vi "Read Coords.vi"(8 "error in (no error)":errorcluster, 11 "ShortcutMenuSelectionMsg in":refnum<class "ShortcutMenuSelectionMsg.lvclass">) -> (0 "error out":errorcluster, 2 "Coords":T1, 3 "ShortcutMenuSelectionMsg out":refnum<class "ShortcutMenuSelectionMsg.lvclass">)   [LabVIEW 2015, in "ActorEvents.lvlib" / "ShortcutMenuSelectionMsg.lvclass"]
uses:
  ShortcutMenuSelectionMsg.lvclass
  <vilib>/Utility/miscctls.llb/LVPoint32TypeDef.ctl
  ShortcutMenuSelectionMsg.lvclass/ShortcutMenuSelectionMsg.ctl
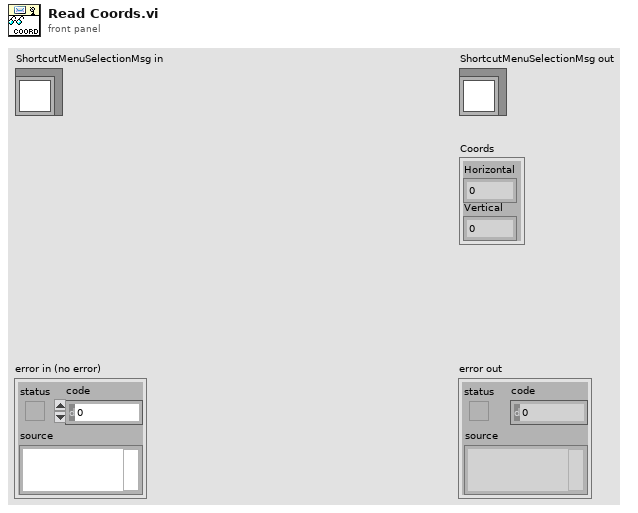
[diagram p1: front panel]
types:
  T1 = typedef "LVPoint32TypeDef.ctl" = cluster{"Horizontal":i32, "Vertical":i32}
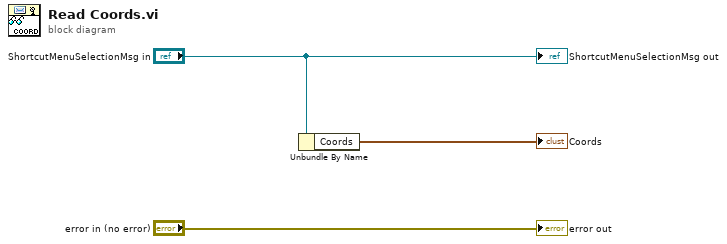
[diagram p0: block diagram]
diagram:
  n1 = Unbundle By Name("ShortcutMenuSelectionMsg in") -> ("Coords"=→"Coords":T1)
  "error out" <- "error in (no error)"
  "ShortcutMenuSelectionMsg out" <- "ShortcutMenuSelectionMsg in"
